vi "DistributePixels2D.vi"(8 "error in (no error)":errorcluster, 10 "Parameters":T1={"number of planes"=4, "z step"=1.9999999999999998e-05, "pixel dwell time"=1.0000000000000001e-11, "z frequency"=10.0, "number of pixels"=100, "smooth points"=10, "smooth line"=10, "Sine\nSawtooth"=FALSE, "PointSorting"=0, "Sort Points"=FALSE, "X-pixels"=256.0, "Y-lines"=256.0, "pixelstoµm"=256.0, "zoom"=1.0, "Time offset"=1.0000000000000001e-11} {"zoom" min=0.5 step=0.1; "Y-lines" min=1 step=1; "X-pixels" min=1 step=1; "PointSorting" items=["No Difference", "Every Second Point", "Down / Up"]; "smooth line" min=1; "smooth points" min=1; "number of pixels" min=1; "z frequency" format="%_4g"; "number of planes" min=1}, 11 "XY coordinates":dbl[][](array[numeric])) -> (0 "error out":errorcluster, 3 "XY coordinates interpolated":dbl[][](array[numeric]))   [LabVIEW 2010]
uses:
  TypeDefs/ParameterCluster.ctl
  <vilib>/Analysis/_algsub.llb/Real Vector Norm.vi
  <vilib>/Analysis/NI_AALPro.lvlib
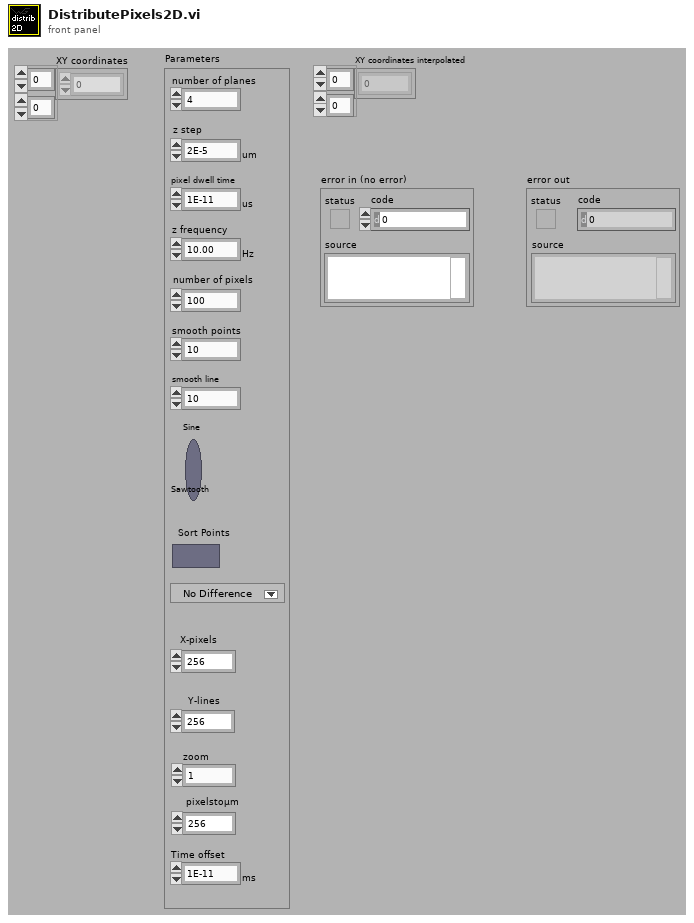
[diagram p1: front panel]
types:
  T1 = typedef "ParameterCluster.ctl" = cluster{"number of planes":i32, "z step":dbl[unit], "pixel dwell time":dbl[unit], "z frequency":dbl[unit], "number of pixels":i32, "smooth points":i32, "smooth line":i32, "Sine\nSawtooth":bool, "PointSorting":u16, "Sort Points":bool, "X-pixels":sgl, "Y-lines":sgl, "pixelstoµm":dbl, "zoom":dbl, "Time offset":dbl[unit]}
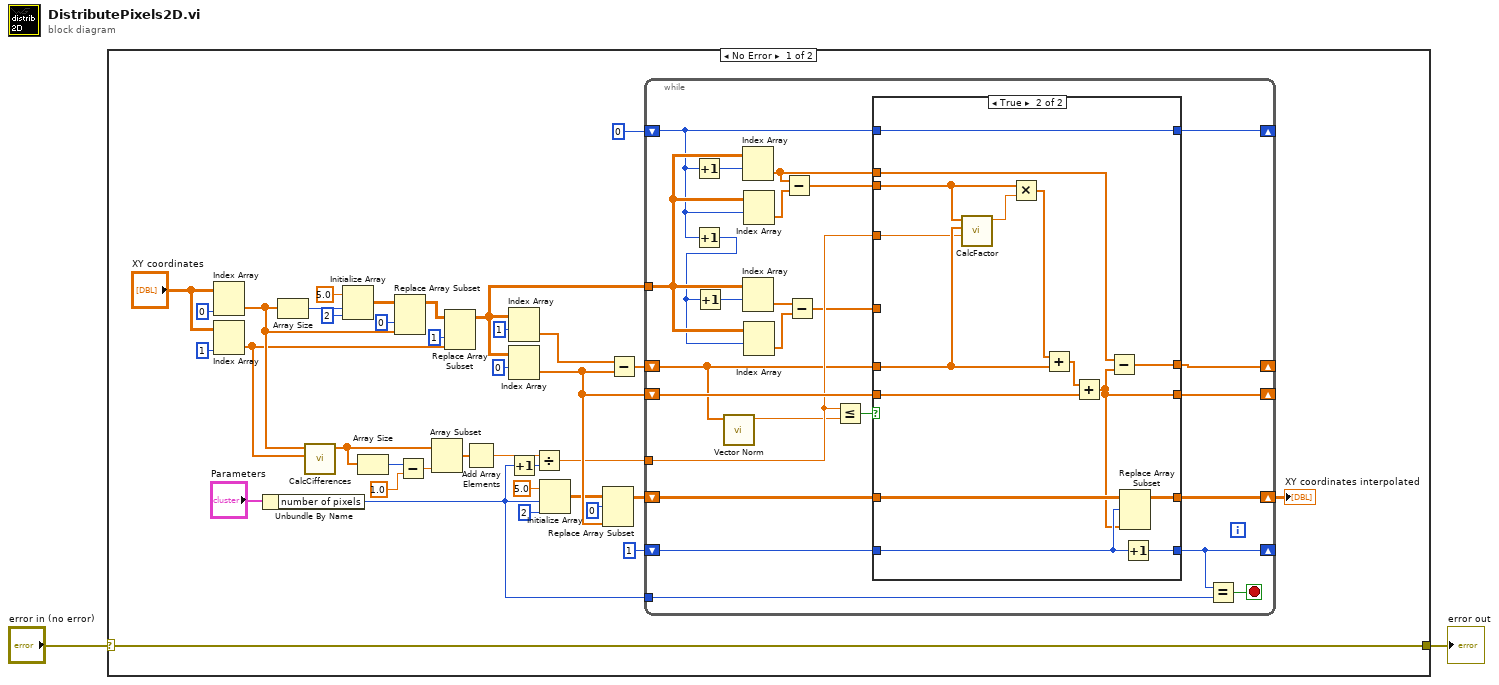
[diagram p0: block diagram]
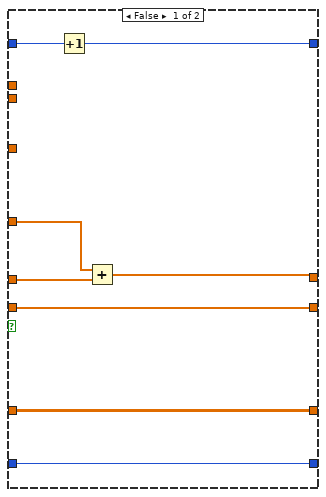
[diagram p2: hidden frame]
diagram:
  n1 = case shown="No Error" "error in (no error)" {
    selector: "error in (no error)" -> [w3 w88]
    tunnel: [w3 w88] -> w1
    frame No Error {
      n2 = Index Array(array="XY coordinates", index (col)=0 ("disabled index (col)")) -> (element=w5:dbl[])  [unwired: 1 in]
      n3 = Index Array(array="XY coordinates", index (col)=1 ("disabled index (col)")) -> (element=w4:dbl[])  [unwired: 1 in]
      n4 = Unbundle By Name("Parameters") -> ("number of pixels"=w9:i32)
      n5 = Array Size(array=w5) -> (size(s)=w33:i32)
      n6 = call "CalcCifferences.vi"("y scan signals UDL"=w4, "x scan signals UDL"=w5) -> ("difference"=w13:dbl[])  [unwired: 8 in, 1 out]
      n7 = Initialize Array(5.0 ("element"), w33, 2 ("dimension size")) -> (w37:dbl[][])
      n8 = Array Size(array=w13) -> (size(s)=w15:i32)
      n9 = Replace Array Subset(array=w37, new element=w5, index (col)=0 ("disabled index (col)")) -> (w35:dbl[][])  [unwired: 1 in]
      n10 = Subtract(x=w15, y=1.0) -> (x-y=w14:dbl)
      n11 = Array Subset(array=w13, length=w14) -> (w12:dbl[])  [unwired: 1 in]
      n12 = Replace Array Subset(array=w35, new element=w4, index (col)=1 ("disabled index (col)")) -> (w17:dbl[][])  [unwired: 1 in]
      n13 = Add Array Elements(numeric array=w12) -> (sum=w28:dbl)
      n14 = Index Array(array=w17, index (row)=1) -> (element=w29:dbl[])  [unwired: 1 in]
      n15 = Index Array(array=w17, index (row)=0) -> (element=w32:dbl[])  [unwired: 1 in]
      n16 = Increment(x=w9) -> (x+1=w11:i32)
      n17 = Divide(x=w28, y=w11) -> (x/y=w24:dbl)
      n18 = Initialize Array(5.0 ("element"), w9, 2 ("dimension size")) -> (w25:dbl[][])
      n19 = Replace Array Subset(array=w25, new element=w32, index (row)=0) -> (w22:dbl[][])  [unwired: 1 in]
      n20 = Subtract(x=w29, y=w32) -> (x-y=w19:dbl[])
      n21 = while {
        tunnel: w17 -> [w46]
        tunnel: w24 -> [w58]
        shift-right: [w62] -> _
        shift-left: w32 -> [w63]
        shift-right: [w64] -> _
        shift-left: w19 -> [w41]
        shift-right: [w56] -> _
        shift-left: 1 -> [w61]
        shift-right: [w44] -> w18
        shift-left: w22 -> [w60]
        shift-right: [w59] -> _
        shift-left: 0 -> [w43]
        tunnel: w9 -> [w42]
        stop <- w57 stop-if-true
        n22 = Increment(x=w43) -> (x+1=w54:i32)
        n23 = Increment(x=w43) -> (x+1=w45:i32)
        n24 = Increment(x=w45) -> (x+1=w51:i32)
        n25 = call-poly <vilib>:"Vector Norm.vi"("Input Vector"=w41) -> ("norm"=w40:dbl)  [unwired: 9 in, 1 out]
        n26 = Index Array(array=w46, index (row)=w54) -> (element=w47:dbl[])  [unwired: 1 in]
        n27 = Index Array(array=w46, index (row)=w51) -> (element=w50:dbl[])  [unwired: 1 in]
        n28 = Index Array(array=w46, index (row)=w43) -> (element=w55:dbl[])  [unwired: 1 in]
        n29 = Index Array(array=w46, index (row)=w45) -> (element=w52:dbl[])  [unwired: 1 in]
        n30 = Subtract(x=w47, y=w55) -> (x-y=w48:dbl[])
        n31 = Subtract(x=w50, y=w52) -> (x-y=w49:dbl[])
        n32 = Less Or Equal?(x=w58, y=w40) -> (x <= y?=w53:bool)
        n33 = case shown="True" w53 {
          tunnel: w41 -> [w67 w75]
          tunnel: w49 -> [w66 _]
          tunnel: [w71 w86] -> w64
          tunnel: w48 -> [_ w73]
          tunnel: w63 -> [w70 w87]
          tunnel: [w70 w76] -> w62
          tunnel: w61 -> [w69 w84]
          tunnel: w60 -> [w68 w85]
          tunnel: [w69 w83] -> w56
          tunnel: [w68 w77] -> w44
          tunnel: w43 -> [w65 w82]
          tunnel: [w72 w82] -> w59
          tunnel: w58 -> [_ w74]
          tunnel: w47 -> [_ w79]
          frame False {
            n34 = Increment(x=w65) -> (x+1=w72:i32)
            n35 = Add(x=w66, y=w67) -> (x+y=w71:dbl[])
          }
          frame True {
            n36 = call "CalcFactor.vi"("delta"=w74, "deltavec"=w75, "point"=w73) -> ("factor"=w78:dbl)  [unwired: 5 in, 1 out]
            n37 = Multiply(x=w73, y=w78) -> (x*y=w80:dbl[])
            n38 = Add(x=w80, y=w75) -> (x+y=w81:dbl[])
            n39 = Add(x=w81, y=w87) -> (x+y=w76:dbl[])
            n40 = Subtract(x=w79, y=w76) -> (x-y=w86:dbl[])
            n41 = Replace Array Subset(array=w85, new element=w76, index (row)=w84) -> (w77:dbl[][])  [unwired: 1 in]
            n42 = Increment(x=w84) -> (x+1=w83:i32)
          }
        }
        n43 = Equal?(x=w56, y=w42) -> (x = y?=w57:bool)
      }
      "XY coordinates interpolated" <- w18
    }
    frame Error {
    }
  }
  "error out" <- w1
